vi "Items to path array.vi"(10 "Project Items":refnum<vi>[](array[refnum])) -> (2 "Paths":path[](array[path]))   [LabVIEW 2019, in "TestRunner.lvlib" / "TestRunner.lvclass"]
uses:
  TestRunner.lvclass
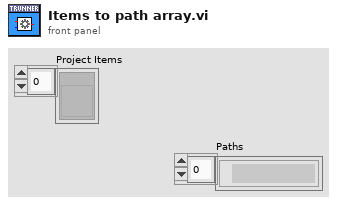
[diagram p1: front panel]
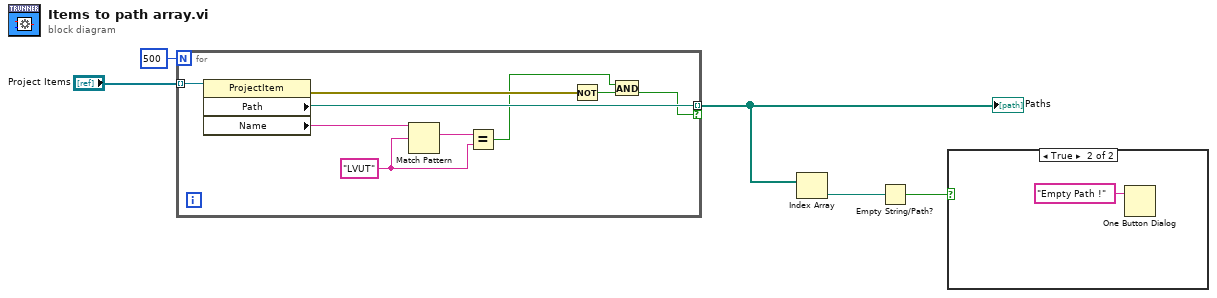
[diagram p0: block diagram]
diagram:
  n1 = for {
    N: 500 -> [_]
    tunnel: "Project Items" -> [w14] mode=indexing
    tunnel: [w13] -> w3 mode=indexing if=w7
    w8 = "LVUT" ("regular expression")
    n2 = property class="ProjectItem"(reference=w14) -> (error out=w12:errorcluster, "Path"=w13:path, "Name"=w10:string)  [unwired: 1 in, 1 out]
    n3 = Match Pattern(string=w10, regular expression=w8) -> (match substring=w9:string)  [unwired: 1 in, 3 out]
    n4 = Equal?(x=w9, y=w8) -> (x = y?=w6:bool)
    n5 = Not(x=w12) -> (.not. x?=w11:bool)
    n6 = And(x=w6, y=w11) -> (x .and. y?=w7:bool)
  }
  "Paths" <- w3
  n7 = Index Array(array=w3) -> (element=w2:path)  [unwired: 1 in]
  n8 = Empty String/Path?(string/path=w2) -> (empty?=w1:bool)
  n9 = case shown="True" w1 {
    frame False {
    }
    frame True {
      n10 = One Button Dialog(message="Empty Path !") -> ()  [unwired: 1 in, 1 out]
    }
  }
